vi "Transform3d_GetXYZ.vi"(11 "inTransform3d":T1={"TRANSLATION3D"={"X"=0.0, "Y"=0.0, "Z"=0.0}, "ROTATION3D"={"Q_quaternion"={"R"=1.0, "V"=[0.0, 0.0, 0.0]}}, "XF"=FALSE} {"TRANSLATION3D"."Z" format="%14.3f"; "TRANSLATION3D"."Y" format="%14.3f"; "TRANSLATION3D"."X" format="%14.3f"}) -> (1 "Z":dbl format="%14.3f", 2 "Y":dbl format="%14.3f", 3 "X":dbl format="%14.3f")   [LabVIEW 2019, in "Trajectory_Library.lvlib"]
doc: "Returns the X, Y, Z elements of the translation3d component of the transformation3d.\n\nParameters:\n - IN TRANSFORM3d -- THis TRANSFORM data structure\n\nReturns:\n - X - The X element of the translational component of the transform.\n - Y - The Y element of the translational component of the transform.\n - Z - The Z element of the translational component of the transform."
uses:
  Trajectory_Library.lvlib
  TypeDef/TRANSLATION3D.ctl
  TypeDef/QUATERNION.ctl
  TypeDef/ROTATION3D.ctl
  TypeDef/TRANSFORM3D.ctl
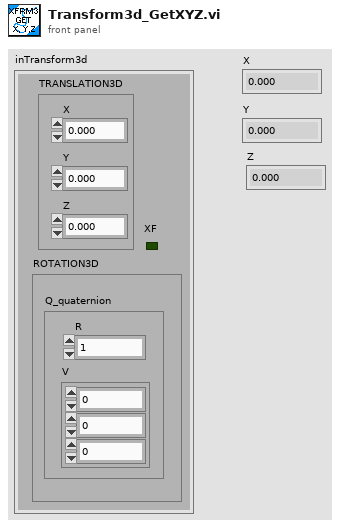
[diagram p1: front panel]
types:
  T1 = typedef "Trajectory_Library.lvlib/TRANSFORM3D.ctl" = cluster{"TRANSLATION3D":T2, "ROTATION3D":T3, "XF":bool}
  T2 = typedef "Trajectory_Library.lvlib/TRANSLATION3D.ctl" = cluster{"X":dbl, "Y":dbl, "Z":dbl}
  T3 = typedef "Trajectory_Library.lvlib/ROTATION3D.ctl" = cluster{"Q_quaternion":T4}
  T4 = typedef "Trajectory_Library.lvlib/QUATERNION.ctl" = cluster{"R":dbl, "V":dbl[]}
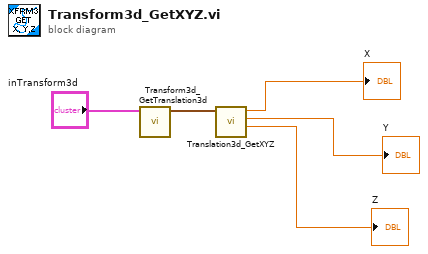
[diagram p0: block diagram]
diagram:
  n1 = call "Transform3d_GetTranslation3d.vi"("in Transform3d"="inTransform3d") -> ("Translation3d"=w4:T2)  [unwired: 10 in]
  n2 = call "Translation3d_GetXYZ.vi"("In Translation3d"=w4) -> ("Z"=→"Z":dbl, "Y"=→"Y":dbl, "X"=→"X":dbl)  [unwired: 8 in]
